vi "Digital Demod Trace LimitY Configure List Data.vi"(6 "TraceLimitType (Upper)":i32(ring) items=["Upper", "Lower"], 7 "ListData":dbl[](array[numeric]) format="%.2p", 8 "error in (no error)":errorcluster {"code" format="%.0x"}, 9 "ListDataBufferSize":i32=2048, 10 "DigitalDemodTraceLimit":string="TraceLimit1", 11 "instrument handle":refnum<k15>) -> (0 "error out":errorcluster {"code" format="%.0x"}, 3 "instrument handle out":refnum<k15>)   [LabVIEW 2021, in "Keysight XSAnVMA.lvlib"]
doc: "Configure a list of y values for selected limit line."
uses:
  <instrlib>/Keysight XSAnVMA/Keysight XSAnVMA.lvlib
  KtXSAnVMA_64.dll
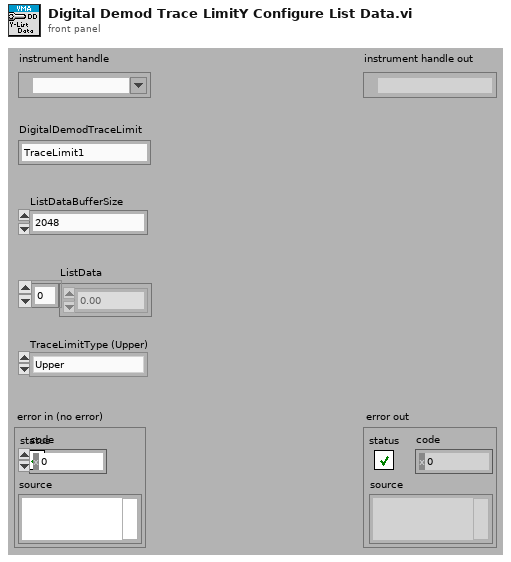
[diagram p1: front panel]
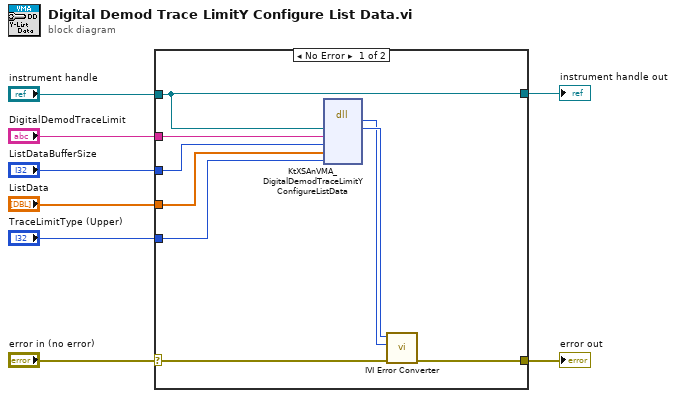
[diagram p0: block diagram]
diagram:
  n1 = case shown="No Error" "error in (no error)" {
    selector: "error in (no error)" -> [w15 w19]
    tunnel: [w14 w19] -> w8
    tunnel: "instrument handle" -> [w9 w18]
    tunnel: "DigitalDemodTraceLimit" -> [w13 _]
    tunnel: "ListDataBufferSize" -> [w12 _]
    tunnel: "ListData" -> [w11 _]
    tunnel: "TraceLimitType (Upper)" -> [w10 _]
    tunnel: [w9 w18] -> w1
    frame No Error {
      n2 = dll-call lib="KtXSAnVMA**.dll" fn="KtXSAnVMA_DigitalDemodTraceLimitYConfigureListData"("Vi"=w9, "DigitalDemodTraceLimit"=w13, "ListDataBufferSize"=w12, "ListData"=w11, "TraceLimitType"=w10) -> (w16:i32, "Vi"=w17:u32)  [unwired: 7 in, 2 out]
      n3 = call <instrlib>:"IVI Error Converter.vi"("error in (no error)"=w15, "IVI error code (0)"=w16, "instrument handle"=w17) -> ("error out"=w14:errorcluster)  [unwired: 7 in, 1 out]
    }
    frame Error {
    }
  }
  "error out" <- w8
  "instrument handle out" <- w1
